vi "Quantizer (DBL).vi"(2 "quantization interval":dbl=0.1 format="%.2f", 3 "input point":dbl format="%.2f") -> (1 "output point":dbl format="%.2f")   [LabVIEW 2020, in "NI_AdvCtrl_nonlinear.lvlib"]
doc: "LabVIEW no longer supports this VI. You can obtain similar functionality by installing the LabVIEW Simulation Module.\n\nQuantizes an input signal. It is output=[input/quantization interval]*quantization interval."
uses:
  <vilib>/addons/control/advanced/NI_AdvCtrl_nonlinear.lvlib
  <vilib>/addons/control/advanced/NI_AdvCtrl_continuous linear.lvlib
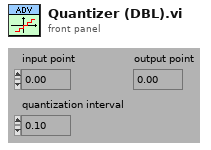
[diagram p1: front panel]
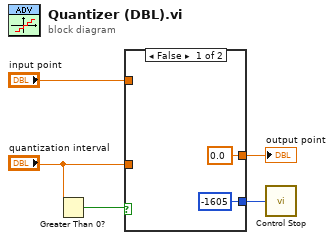
[diagram p0: block diagram]
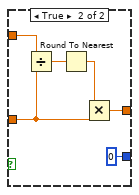
[diagram p2: hidden frame]
diagram:
  n1 = Greater Than 0?(x="quantization interval") -> (x > 0?=w2:bool)
  n2 = case shown="False" w2 {
    tunnel: [0.0 w13] -> w5
    tunnel: "input point" -> [_ w10]
    tunnel: "quantization interval" -> [_ w9]
    tunnel: [-1605 ("error") 0 ("error")] -> w1
    frame False {
    }
    frame True {
      n3 = Divide(x=w10, y=w9) -> (x/y=w11:dbl)
      n4 = Round To Nearest(number=w11) -> (nearest integer value=w12:dbl)
      n5 = Multiply(x=w12, y=w9) -> (x*y=w13:dbl)
    }
  }
  "output point" <- w5
  n6 = call <vilib>:"Control Stop.vi"("error"=w1) -> ()  [unwired: 2 out]
